vi "IDW Combined Format - Multi Byte.vi"() -> ()   [LabVIEW 2009]
doc: "An example program for the I2C Digital Waveform library. This VI constructs a simple master combined-format waveform for a multi-byte write/read operation on an I2C bus."
uses:
  user.lib/I2C Digital Waveform/_Typedefs/Timing - ns.ctl
  user.lib/I2C Digital Waveform/_Typedefs/Bus mode.ctl
  user.lib/I2C Digital Waveform/_Typedefs/Bit type.ctl
  user.lib/I2C Digital Waveform/_Polymorphics/Init - Preallocate.vi
  user.lib/I2C Digital Waveform/_Typedefs/Bus operation.ctl
  user.lib/I2C Digital Waveform/_Typedefs/Start action.ctl
  user.lib/I2C Digital Waveform/_Typedefs/ACK action.ctl
  user.lib/I2C Digital Waveform/IDW.lvlib
panel:
  out "Compare bits":cluster{"Locations":u64[], "Types":T1[]}
  in  "Sample quantum (min 1)":i32=2 caption="Sample quantum\n(min 1)" min=1
  in  "Tx data":u8[](array[numeric])=[1, 35, 69, 103] format="%02x"
  in  "Samples to allocate":i32=100000 format="%.0p"
  out "Coerced timing (ns)":T2 {"fSCL" format="%#_6p"}
  out "I2C digital waveform":digitalwaveform(graph)
  in  "Sample rate":dbl=100000000.0 format="%#_6p"
  in  "Mode":T3="Standard-mode"
  in  "I2C timing (ns)":T2={"tSU;STA"=4700, "tHD;STA"=4000, "tSU;DAT"=250, "tHD;DAT"=5000, "tSU;STO"=4000, "tBUF"=4700, "tHIGH"=4000, "fSCL"=100000.0} {"fSCL" format="%#_6p"}
  in  "Expected Rx data":u8[](array[numeric])=[1, 35, 69, 103] format="%02x"
  in  "Slave address":u8=170 format="%02x"
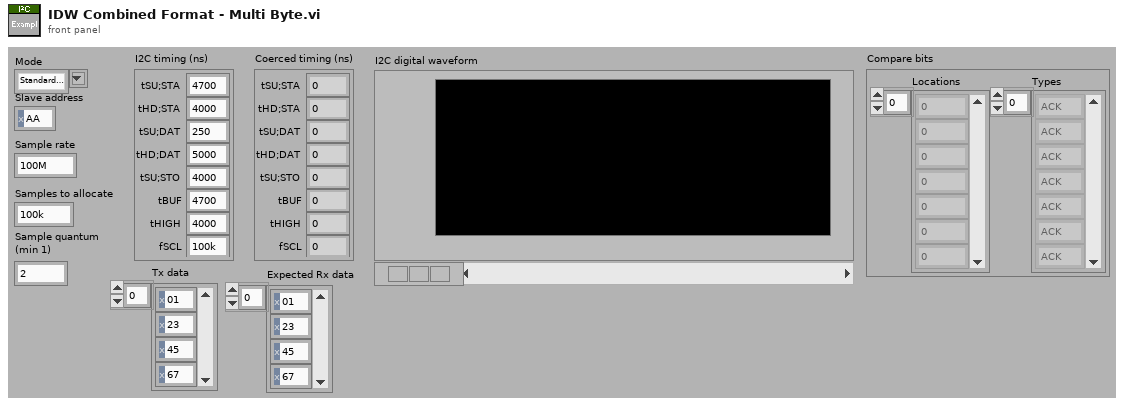
[diagram p1: front panel]
types:
  T1 = typedef "IDW.lvlib/Bit type.ctl" = enum16{"ACK", "Data"}
  T2 = typedef "IDW.lvlib/Timing - ns.ctl" = cluster{"tSU;STA":i32, "tHD;STA":i32, "tSU;DAT":i32, "tHD;DAT":i32, "tSU;STO":i32, "tBUF":i32, "tHIGH":i32, "fSCL":dbl}
  T3 = typedef "IDW.lvlib/Bus mode.ctl" = string
  T4 = cluster{"tSU;STA":bool, "tHD;STA":bool, "tSU;DAT":bool, "tHD;DAT":bool, "tSU;STO":bool, "tBUF":bool, "tHIGH":bool, "fSCL":bool}
  T5 = typedef "IDW.lvlib/Start action.ctl" = enum16{"S", "Sr"}
  T6 = typedef "IDW.lvlib/ACK action.ctl" = enum16{"Listen ACK", "Listen NACK", "Send ACK", "Send NACK"}
  T7 = typedef "IDW.lvlib/Bus operation.ctl" = enum16{"Tx", "Rx"}
  T8 = typedef "IDW.lvlib/Waveform info.ctl" = cluster{"Last sample":u8[], "Sample offset":u64, "Compare offset":u64, "Timing (ticks)":T9, "Preallocated":bool, "Def trans action":T10, "Data Q":refnum<queue>, "Comp types Q":refnum<queue>, "Comp locs Q":refnum<queue>}
  T9 = typedef "IDW.lvlib/Timing - ticks.ctl" = cluster{"tSU;STA":i32, "tHD;STA":i32, "tSU;DAT":i32, "tHD;DAT":i32, "tSU;STO":i32, "tBUF":i32, "tHIGH":i32, "Trans length":i32, "0-30 Rise":i32, "0-70 Rise":i32, "100-30 Fall":i32}
  T10 = typedef "IDW.lvlib/Default transition action.ctl" = enum16{"Hold low (0)", "Release (Z)", "Set up next value", "Hold previous value", "Preserve tHD;DAT and tSU;DAT"}
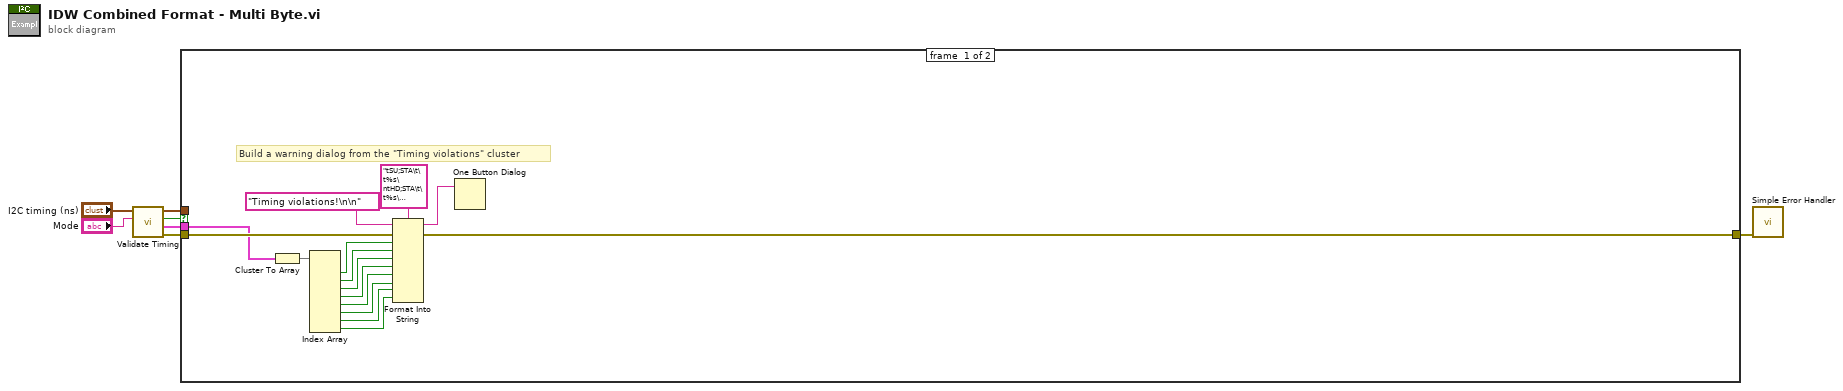
[diagram p0: block diagram]
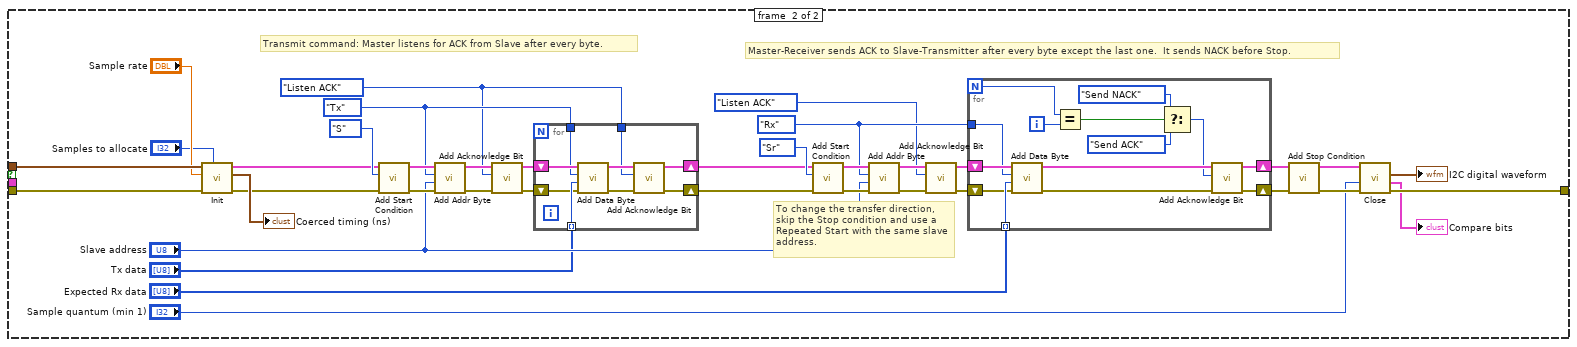
[diagram p2: hidden frame]
diagram:
  n1 = call "Validate Timing.vi"("Mode"="Mode", "I2C timing (ns)"="I2C timing (ns)") -> ("error out"=w2:errorcluster, "Timing violations"=w3:T4, "Timing passed?"=w4:bool, "I2C timing (ns) out"=w7:T2)  [unwired: 1 in, 5 out]
  n2 = case shown="True" w4 {
    tunnel: w7 -> [_ w45]
    tunnel: w3 -> [w9 _]
    tunnel: w2 -> [w10 w42]
    tunnel: [w8 w25] -> w1
    frame #0 {
      # "Build a warning dialog from the \"Timing violations\" cluster"
      n3 = Cluster To Array(cluster=w9) -> (array=w22:bool[])
      n4 = Index Array(array=w22) -> (element #1=w21:bool, element #2=w20:bool, element #3=w19:bool, element #4=w18:bool, element #5=w17:bool, element #6=w16:bool, element #7=w15:bool, element #8=w14:bool)  [unwired: 8 in]
      n5 = Format Into String(format string="tSU;STA\t\t%s\ntHD;STA\t\t%s\ntSU;DAT\t\t%s\ntHD;DAT\t\t%s\ntSU;STO\t\t%s\ntBUF\t\t%s\ntHIGH\t\t%s\nfSCL\t\t%s", initial string="Timing violations!\n\n", error in=w10, w21, w20, w19, w18, w17, w16, w15, w14) -> (resulting string=w11:string, error out=w8:errorcluster)
      n6 = One Button Dialog(message=w11) -> ()  [unwired: 2 out]
    }
    frame #1 {
      w36 = Bus_operation."Tx" ("Bus operation")
      w35 = ACK_action."Listen ACK" ("Action")
      w55 = Bus_operation."Rx" ("Bus operation")
      # "Master-Receiver sends ACK to Slave-Transmitter after every byte except the last one.  It sends NACK before Stop."
      # "To change the transfer direction, skip the Stop condition and use a Repeated Start with the same slave address."
      # "Transmit command: Master listens for ACK from Slave after every byte."
      n7 = call-poly "Init.vi"("Samples to allocate"="Samples to allocate", "error in (no error)"=w42, "Sample rate"="Sample rate", "I2C timing (ns)"=w45) -> ("error out"=w31:errorcluster, "Coerced I2C timing (ns)"=→"Coerced timing (ns)":T2, "I2C waveform info"=w30:T8)  [unwired: 1 in, 4 out]
      n8 = call "Add Start Condition.vi"("error in (no error)"=w31, "Action"=Start_action."S", "I2C waveform info"=w30) -> ("error out"=w34:errorcluster, "I2C waveform info out"=w40:T8)  [unwired: 1 in, 6 out]
      n9 = call "Add Addr Byte.vi"("error in (no error)"=w34, "Slave address"="Slave address", "Bus operation"=w36, "I2C waveform info"=w40) -> ("error out"=w33:errorcluster, "I2C waveform info out"=w39:T8)  [unwired: 6 out]
      n10 = call "Add Acknowledge Bit.vi"("error in (no error)"=w33, "Action"=w35, "I2C waveform info"=w39) -> ("error out"=w32:errorcluster, "I2C waveform info out"=w38:T8)  [unwired: 7 out]
      n11 = for {
        tunnel: "Tx data" -> [w66] mode=indexing
        tunnel: w36 -> [w65]
        tunnel: w35 -> [w64]
        shift-right: [w67] -> w29
        shift-left: w38 -> [w69]
        shift-right: [w61] -> w28
        shift-left: w32 -> [w63]
        n12 = call "Add Data Byte.vi"("error in (no error)"=w63, "Data"=w66, "Action"=w65, "I2C waveform info"=w69) -> ("error out"=w62:errorcluster, "I2C waveform info out"=w68:T8)  [unwired: 6 out]
        n13 = call "Add Acknowledge Bit.vi"("error in (no error)"=w62, "Action"=w64, "I2C waveform info"=w68) -> ("error out"=w61:errorcluster, "I2C waveform info out"=w67:T8)  [unwired: 7 out]
      }
      n14 = call "Add Start Condition.vi"("error in (no error)"=w28, "Action"=Start_action."Sr", "I2C waveform info"=w29) -> ("error out"=w51:errorcluster, "I2C waveform info out"=w60:T8)  [unwired: 1 in, 6 out]
      n15 = call "Add Addr Byte.vi"("error in (no error)"=w51, "Slave address"="Slave address", "Bus operation"=w55, "I2C waveform info"=w60) -> ("error out"=w50:errorcluster, "I2C waveform info out"=w59:T8)  [unwired: 6 out]
      n16 = call "Add Acknowledge Bit.vi"("error in (no error)"=w50, "Action"=ACK_action."Listen ACK", "I2C waveform info"=w59) -> ("error out"=w49:errorcluster, "I2C waveform info out"=w58:T8)  [unwired: 7 out]
      n17 = for {
        N -> [w74]
        tunnel: "Expected Rx data" -> [w80] mode=indexing
        tunnel: w55 -> [w79]
        shift-right: [w81] -> w57
        shift-left: w58 -> [w83]
        shift-right: [w76] -> w48
        shift-left: w49 -> [w78]
        i -> [w75]
        n18 = call "Add Data Byte.vi"("error in (no error)"=w78, "Data"=w80, "Action"=w79, "I2C waveform info"=w83) -> ("error out"=w77:errorcluster, "I2C waveform info out"=w82:T8)  [unwired: 6 out]
        n19 = Equal?(x=w74, y=w75) -> (x = y?=w73:bool)
        n20 = Select(t=ACK_action."Send NACK" ("Action"), s=w73, f=ACK_action."Send ACK" ("Action")) -> (s? t:f=w70:T6)
        n21 = call "Add Acknowledge Bit.vi"("error in (no error)"=w77, "Action"=w70, "I2C waveform info"=w82) -> ("error out"=w76:errorcluster, "I2C waveform info out"=w81:T8)  [unwired: 7 out]
      }
      n22 = call "Add Stop Condition.vi"("error in (no error)"=w48, "I2C waveform info"=w57) -> ("error out"=w47:errorcluster, "I2C waveform info out"=w53:T8)  [unwired: 8 out]
      n23 = call "Close.vi"("error in (no error)"=w47, "Sample quantum (min 1)"="Sample quantum (min 1)", "I2C waveform info"=w53) -> ("error out"=w25:errorcluster, "Compare bits"=→"Compare bits":cluster{"Locations":u64[], "Types":T1[]}, "Dig waveform out"=→"I2C digital waveform":digitalwaveform)  [unwired: 1 in, 5 out]
    }
  }
  n24 = call <vilib>:"Simple Error Handler.vi"("error in (no error)"=w1) -> ()  [unwired: 1 in, 8 out]
